vi "RampToSetpoint.vi"(8 "error in (no error)":errorcluster, 11 "PS Control Actor in":refnum<class "PS Control Actor.lvclass">) -> (0 "error out":errorcluster, 3 "PS Control Actor out":refnum<class "PS Control Actor.lvclass">)   [LabVIEW 2019, in "PS Control Actor.lvlib" / "PS Control Actor.lvclass"]
uses:
  PS Control Actor.lvclass
  PS Control Actor.lvclass/PS Control Actor.ctl
  PS Driver/PS Driver.lvclass
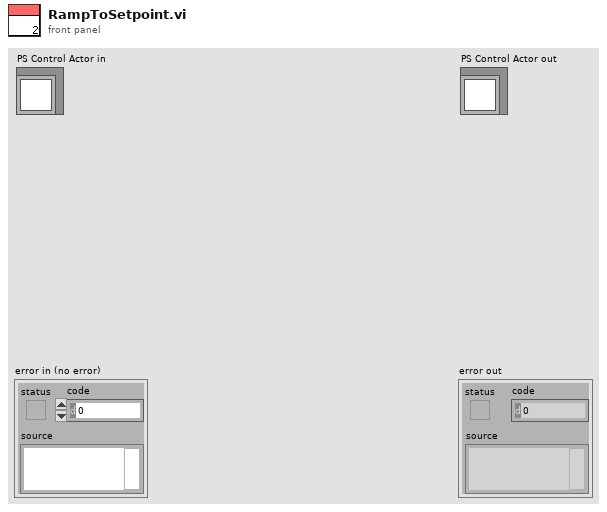
[diagram p1: front panel]
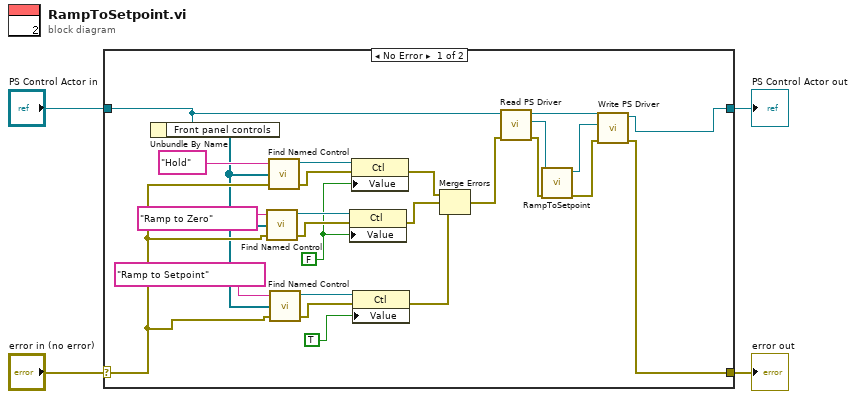
[diagram p0: block diagram]
diagram:
  n1 = case shown="No Error" "error in (no error)" {
    selector: "error in (no error)" -> [w16 w31]
    tunnel: [w10 w31] -> w3
    tunnel: [w11 w30] -> w1
    tunnel: "PS Control Actor in" -> [w13 w30]
    frame No Error {
      w21 = FALSE
      n2 = Unbundle By Name(w13) -> ("Front panel controls"=w15:refnum<vi>[])
      n3 = call "Find Named Control.vi"("error in"=w16, "All Controls"=w15, "Control Name"="Ramp to Zero") -> ("error out"=w25:errorcluster, "Ctl Refnum"=w26:refnum<vi>)  [unwired: 1 out]
      n4 = call "Find Named Control.vi"("error in"=w16, "All Controls"=w15, "Control Name"="Hold") -> ("error out"=w28:errorcluster, "Ctl Refnum"=w29:refnum<vi>)  [unwired: 1 out]
      n5 = call "Find Named Control.vi"("error in"=w16, "All Controls"=w15, "Control Name"="Ramp to Setpoint") -> ("error out"=w19:errorcluster, "Ctl Refnum"=w20:refnum<vi>)  [unwired: 1 out]
      n6 = property class="Ctl"(reference=w26, error in=w25, "Value"=w21) -> (error out=w22:errorcluster)  [unwired: 1 out]
      n7 = property class="Ctl"(reference=w29, error in=w28, "Value"=w21) -> (error out=w23:errorcluster)  [unwired: 1 out]
      n8 = property class="Ctl"(reference=w20, error in=w19, "Value"=TRUE) -> (error out=w14:errorcluster)  [unwired: 1 out]
      n9 = Merge Errors(w23, w22, w14) -> (w7:errorcluster)
      n10 = call-dynamic "Read PS Driver.vi"("error in (no error)"=w7, "PS Control Actor in"=w13) -> ("error out"=w8:errorcluster, "PS Driver.lvlib:PS Driver.lvclass"=w6:refnum<class "PS Driver.lvclass">, "PS Control Actor out"=w12:refnum<class "PS Control Actor.lvclass">)  [unwired: 7 in]
      n11 = call-dynamic "RampToSetpoint.vi"("error in (no error)"=w8, "PS Driver.lvlib:PS Driver.lvclass in"=w6) -> ("error out"=w9:errorcluster, "PS Driver.lvlib:PS Driver.lvclass out"=w5:refnum<class "PS Driver.lvclass">)  [unwired: 8 in]
      n12 = call-dynamic "Write PS Driver.vi"("error in (no error)"=w9, "PS Driver.lvlib:PS Driver.lvclass"=w5, "PS Control Actor in"=w12) -> ("error out"=w10:errorcluster, "PS Control Actor out"=w11:refnum<class "PS Control Actor.lvclass">)  [unwired: 7 in]
    }
    frame Error {
    }
  }
  "error out" <- w3
  "PS Control Actor out" <- w1
